vi "XIPIN_DDR3_and_DDR4_PHY_IP_1_2.vi"   [LabVIEW 2017]
doc: "PHY for DDR3 and DDR4 interfaces for Ultrascale Architecture\n------------------------------------\n<b>Need License</b> : No"
uses:
  <vilib>/rvi/XilinxIP/XIPIN_XNode/niFpgaXIPIN.xnode
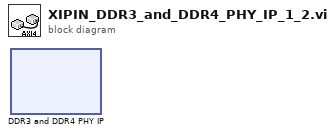
[diagram p0: block diagram]
diagram:
  n1 = xnode ("DDR3 and DDR4 PHY IP")() -> ()
